vi "Set_Source_Library_Data.vi"(8 "error in (no error)":errorcluster, 10 "data":T1, 11 "Class in":refnum<class "AB_Source_Library.lvclass">) -> (0 "error out":errorcluster, 3 "Class out":refnum<class "AB_Source_Library.lvclass">)   [LabVIEW 2020, in "AB_Source_Library.lvclass"]
uses:
  <vilib>/AppBuilder/AB_Classes/Source/Library/AB_Source_Library.lvclass
  <vilib>/AppBuilder/AB_Classes/Source/Library/AB_Source_Library.ctl
  <vilib>/AppBuilder/AB_Classes/Source/Library/AB_Source_Library.lvclass/AB_Source_Library.ctl
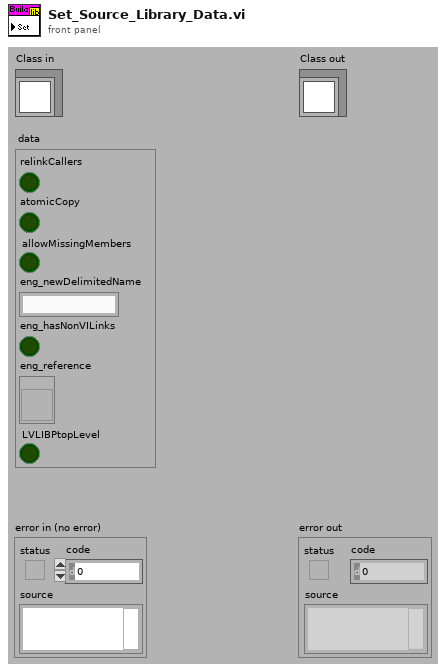
[diagram p1: front panel]
types:
  T1 = typedef "AB_Source_Library.ctl" = cluster{"relinkCallers":bool, "atomicCopy":bool, "allowMissingMembers":bool, "eng_newDelimitedName":string, "eng_hasNonVILinks":bool, "eng_reference":refnum<vi>, "LVLIBPtopLevel":bool}
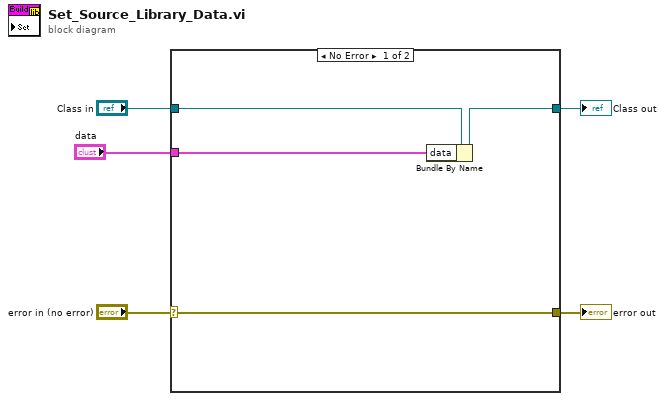
[diagram p0: block diagram]
diagram:
  n1 = case "Case" shown="No Error" "error in (no error)" {
    selector: "error in (no error)" -> [w9 w11]
    tunnel: [w9 w11] -> w4
    tunnel: [w8 w10] -> w2
    tunnel: "Class in" -> [w7 w10]
    tunnel: "data" -> [w6 _]
    frame No Error {
      n2 = Bundle By Name(cluster=w7, "data"=w6) -> (w8:refnum<class "AB_Source_Library.lvclass">)
    }
    frame Error {
    }
  }
  "error out" <- w4
  "Class out" <- w2
